vi "PhotonTrackedTarget_Pack.vi"(11 "TrackedTarget":T1={"Yaw"=0.0, "Pitch"=0.0, "Area"=0.0, "Skew"=0.0, "MinAreaRectCorners"=[], "BestCameraToTarget"={"TRANSLATION3D"={"X"=0.0, "Y"=0.0, "Z"=0.0}, "ROTATION3D"={"Q_quaternion"={"R"=1.0, "V"=[0.0, 0.0, 0.0]}}, "XF"=FALSE}, "FiiducialId"=0, "AltCameraToTarget"={"TRANSLATION3D"={"X"=0.0, "Y"=0.0, "Z"=0.0}, "ROTATION3D"={"Q_quaternion"={"R"=1.0, "V"=[0.0, 0.0, 0.0]}}, "XF"=FALSE}, "PoseAmbiguity"=0.0, "DetectedCorners"=[]} {"AltCameraToTarget"."TRANSLATION3D"."Z" format="%14.3f"; "AltCameraToTarget"."TRANSLATION3D"."Y" format="%14.3f"; "AltCameraToTarget"."TRANSLATION3D"."X" format="%14.3f"; "BestCameraToTarget"."TRANSLATION3D"."Z" format="%14.3f"; "BestCameraToTarget"."TRANSLATION3D"."Y" format="%14.3f"; "BestCameraToTarget"."TRANSLATION3D"."X" format="%14.3f"}) -> (3 "RawData Out":u8[](array[numeric]))   [LabVIEW 2019, in "PhotonVisionLib.lvlib"]
doc: "Encode a TrackedTarget cluster into an array of bytes.\n\nInputs:\n - TrackedTarget -- TrackedTarget cluster.\n\nOutputs:\n - RawDataOut -- Byte array containing the encoded data."
uses:
  PhotonVisionLib.lvlib
  TypeDef/PhotonTrackedTargetType.ctl
  TypeDef/TargetCornerType.ctl
  <vilib>/Rock Robotics/WPI/ThirdParty/JAS_Junk/TrajLib/TypeDef/TRANSFORM3D.ctl
  <vilib>/Rock Robotics/WPI/ThirdParty/JAS_Junk/TrajLib/TypeDef/TRANSLATION3D.ctl
  <vilib>/Rock Robotics/WPI/ThirdParty/JAS_Junk/TrajLib/TypeDef/ROTATION3D.ctl
  <vilib>/Rock Robotics/WPI/ThirdParty/JAS_Junk/TrajLib/TypeDef/QUATERNION.ctl
  <vilib>/Rock Robotics/WPI/ThirdParty/JAS_Junk/TrajLib/VI/Transform3d_GetRotation3d.vi
  <vilib>/Rock Robotics/WPI/ThirdParty/JAS_Junk/TrajLib/VI/Transform3d_GetTranslation3d.vi
  <vilib>/Rock Robotics/WPI/ThirdParty/JAS_Junk/TrajLib/VI/Translation3d_ToTranslation2d.vi
  <vilib>/Rock Robotics/WPI/ThirdParty/JAS_Junk/TrajLib/VI/Rotation3d_ToRotation2d.vi
  <vilib>/Rock Robotics/WPI/ThirdParty/JAS_Junk/TrajLib/Transform2d_Create_TransRot.vi
  <vilib>/Rock Robotics/WPI/ThirdParty/JAS_Junk/TrajLib/VI/Transform3d_GetXYZ.vi
  <vilib>/Rock Robotics/WPI/ThirdParty/JAS_Junk/TrajLib/VI/Rotation3d_GetQuaterion.vi
  <vilib>/Rock Robotics/WPI/ThirdParty/JAS_Junk/TrajLib/VI/Quaternion_Get_All.vi
  <vilib>/Rock Robotics/WPI/ThirdParty/JAS_Junk/TrajLib/Translation2d_Create.vi
  <vilib>/Rock Robotics/WPI/ThirdParty/JAS_Junk/TrajLib/Rotation2d_CreateAngle.vi
  <vilib>/Rock Robotics/WPI/ThirdParty/JAS_Junk/TrajLib/VI/Rotation3d_GetXYZ.vi
  <vilib>/Rock Robotics/WPI/ThirdParty/JAS_Junk/TrajLib/VI/Translation3d_GetXYZ.vi
  <vilib>/Rock Robotics/WPI/ThirdParty/JAS_Junk/TrajLib/Trajectory_Library.lvlib
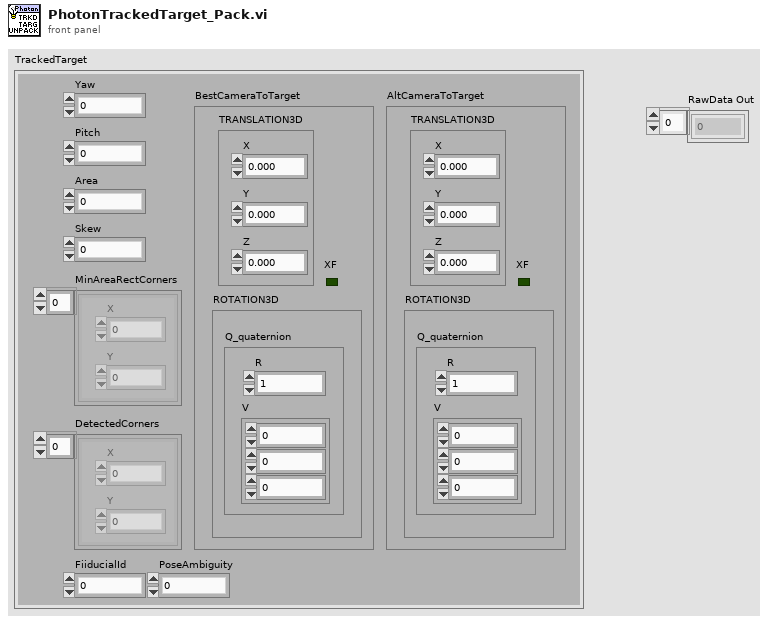
[diagram p1: front panel]
types:
  T1 = typedef "PhotonVisionLib.lvlib/PhotonTrackedTargetType.ctl" = cluster{"Yaw":dbl, "Pitch":dbl, "Area":dbl, "Skew":dbl, "MinAreaRectCorners":T2[], "BestCameraToTarget":T3, "FiiducialId":i32, "AltCameraToTarget":T3, "PoseAmbiguity":dbl, "DetectedCorners":T2[]}
  T2 = typedef "PhotonVisionLib.lvlib/TargetCornerType.ctl" = cluster{"X":dbl, "Y":dbl}
  T3 = typedef "Trajectory_Library.lvlib/TRANSFORM3D.ctl" = cluster{"TRANSLATION3D":T4, "ROTATION3D":T5, "XF":bool}
  T4 = typedef "Trajectory_Library.lvlib/TRANSLATION3D.ctl" = cluster{"X":dbl, "Y":dbl, "Z":dbl}
  T5 = typedef "Trajectory_Library.lvlib/ROTATION3D.ctl" = cluster{"Q_quaternion":T6}
  T6 = typedef "Trajectory_Library.lvlib/QUATERNION.ctl" = cluster{"R":dbl, "V":dbl[]}
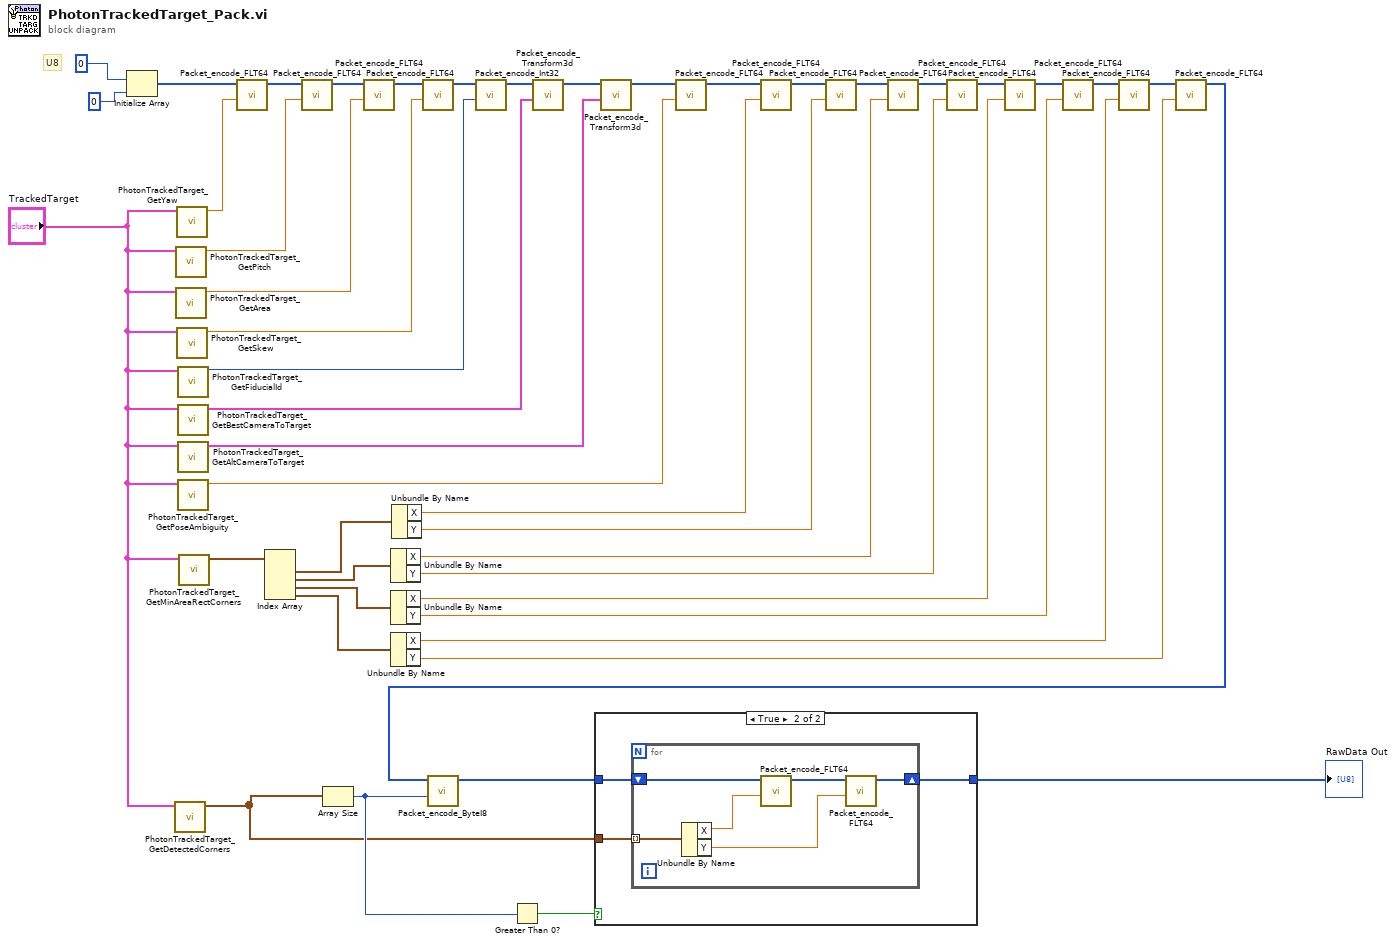
[diagram p0: block diagram]
diagram:
  # "U8"
  n1 = Initialize Array(u8 0 ("element"), 0 ("dimension size")) -> (w44:u8[])
  n2 = call "PhotonTrackedTarget_GetDetectedCorners.vi"("TrackedTarget"="TrackedTarget") -> ("Detected Corners"=w1:T2[])  [unwired: 10 in]
  n3 = call "PhotonTrackedTarget_GetPitch.vi"("TrackedTarget"="TrackedTarget") -> ("Pitch"=w39:dbl)  [unwired: 10 in]
  n4 = call "PhotonTrackedTarget_GetArea.vi"("TrackedTarget"="TrackedTarget") -> ("Area"=w38:dbl)  [unwired: 10 in]
  n5 = call "PhotonTrackedTarget_GetYaw.vi"("TrackedTarget"="TrackedTarget") -> ("Yaw"=w40:dbl)  [unwired: 10 in]
  n6 = call "PhotonTrackedTarget_GetSkew.vi"("TrackedTarget"="TrackedTarget") -> ("Skew"=w37:dbl)  [unwired: 10 in]
  n7 = call "PhotonTrackedTarget_GetFiducialId.vi"("TrackedTarget"="TrackedTarget") -> ("Fiducial Id"=w15:i32)  [unwired: 10 in]
  n8 = call "PhotonTrackedTarget_GetBestCameraToTarget.vi"("TrackedTarget"="TrackedTarget") -> ("BestCameraToTarget"=w9:T3)  [unwired: 9 in, 1 out]
  n9 = call "PhotonTrackedTarget_GetAltCameraToTarget.vi"("TrackedTarget"="TrackedTarget") -> ("AltCameraToTarget"=w8:T3)  [unwired: 9 in, 1 out]
  n10 = call "PhotonTrackedTarget_GetPoseAmbiguity.vi"("TrackedTarget"="TrackedTarget") -> ("Pose Ambiguity"=w14:dbl)  [unwired: 10 in]
  n11 = call "PhotonTrackedTarget_GetMinAreaRectCorners.vi"("TrackedTarget"="TrackedTarget") -> ("MinAreaRectCorners"=w36:T2[])  [unwired: 10 in]
  n12 = call "Packet_encode_FLT64.vi"("FLT64_Value"=w40, "RawData In"=w44) -> ("RawData Out"=w43:u8[])  [unwired: 9 in]
  n13 = Index Array(array=w36) -> (element #1=w35:T2, element #2=w34:T2, element #3=w33:T2, element #4=w32:T2)  [unwired: 4 in]
  n14 = call "Packet_encode_FLT64.vi"("FLT64_Value"=w39, "RawData In"=w43) -> ("RawData Out"=w42:u8[])  [unwired: 9 in]
  n15 = Array Size(array=w1) -> (size(s)=w4:i32)
  n16 = call "Packet_encode_FLT64.vi"("FLT64_Value"=w38, "RawData In"=w42) -> ("RawData Out"=w41:u8[])  [unwired: 9 in]
  n17 = Unbundle By Name(w34) -> ("X"=w22:dbl, "Y"=w21:dbl)
  n18 = Unbundle By Name(w33) -> ("X"=w20:dbl, "Y"=w19:dbl)
  n19 = Unbundle By Name(w32) -> ("X"=w18:dbl, "Y"=w17:dbl)
  n20 = Unbundle By Name(w35) -> ("X"=w24:dbl, "Y"=w23:dbl)
  n21 = call "Packet_encode_FLT64.vi"("FLT64_Value"=w37, "RawData In"=w41) -> ("RawData Out"=w16:u8[])  [unwired: 9 in]
  n22 = call "Packet_encode_Int32.vi"("Int32_Value"=w15, "RawData In"=w16) -> ("RawData Out"=w13:u8[])  [unwired: 9 in]
  n23 = Greater Than 0?(x=w4) -> (x > 0?=w5:bool)
  n24 = call "Packet_encode_Transform3d.vi"("Transform3d Value"=w9, "RawData In"=w13) -> ("RawData Out"=w12:u8[])  [unwired: 9 in]
  n25 = call "Packet_encode_Transform3d.vi"("Transform3d Value"=w8, "RawData In"=w12) -> ("RawData Out"=w11:u8[])  [unwired: 9 in]
  n26 = call "Packet_encode_FLT64.vi"("FLT64_Value"=w14, "RawData In"=w11) -> ("RawData Out"=w10:u8[])  [unwired: 9 in]
  n27 = call "Packet_encode_FLT64.vi"("FLT64_Value"=w24, "RawData In"=w10) -> ("RawData Out"=w31:u8[])  [unwired: 9 in]
  n28 = call "Packet_encode_FLT64.vi"("FLT64_Value"=w23, "RawData In"=w31) -> ("RawData Out"=w30:u8[])  [unwired: 9 in]
  n29 = call "Packet_encode_FLT64.vi"("FLT64_Value"=w22, "RawData In"=w30) -> ("RawData Out"=w29:u8[])  [unwired: 9 in]
  n30 = call "Packet_encode_FLT64.vi"("FLT64_Value"=w21, "RawData In"=w29) -> ("RawData Out"=w28:u8[])  [unwired: 9 in]
  n31 = call "Packet_encode_FLT64.vi"("FLT64_Value"=w20, "RawData In"=w28) -> ("RawData Out"=w27:u8[])  [unwired: 9 in]
  n32 = call "Packet_encode_FLT64.vi"("FLT64_Value"=w19, "RawData In"=w27) -> ("RawData Out"=w26:u8[])  [unwired: 9 in]
  n33 = call "Packet_encode_FLT64.vi"("FLT64_Value"=w18, "RawData In"=w26) -> ("RawData Out"=w25:u8[])  [unwired: 9 in]
  n34 = call "Packet_encode_FLT64.vi"("FLT64_Value"=w17, "RawData In"=w25) -> ("RawData Out"=w6:u8[])  [unwired: 9 in]
  n35 = call "Packet_encode_ByteI8.vi"("Int8_Value"=w4, "RawData In"=w6) -> ("RawData Out"=w3:u8[])  [unwired: 9 in]
  n36 = case shown="True" w5 {
    tunnel: w3 -> [w47 w50]
    tunnel: [w47 w48] -> w2
    tunnel: w1 -> [_ w49]
    frame False {
    }
    frame True {
      n37 = for {
        shift-right: [w51] -> w48
        shift-left: w50 -> [w54]
        tunnel: w49 -> [w55] mode=indexing
        n38 = Unbundle By Name(w55) -> ("X"=w53:dbl, "Y"=w52:dbl)
        n39 = call "Packet_encode_FLT64.vi"("FLT64_Value"=w53, "RawData In"=w54) -> ("RawData Out"=w56:u8[])  [unwired: 9 in]
        n40 = call "Packet_encode_FLT64.vi"("FLT64_Value"=w52, "RawData In"=w56) -> ("RawData Out"=w51:u8[])  [unwired: 9 in]
      }
    }
  }
  "RawData Out" <- w2
